vi "GetDatDisplayNm.vi"(8 "error in (no error)":errorcluster caption="entrée d'erreur (pas d'erreur)", 11 "BaseDevice en entrée":refnum<class "BaseDevice.lvclass">) -> (0 "error out":errorcluster caption="sortie d'erreur", 2 "DatDisplayNm":string[](array[string]), 3 "BaseDevice en sortie":refnum<class "BaseDevice.lvclass">)   [LabVIEW 2019, in "BaseDevice.lvclass"]
uses:
  BaseDevice.lvclass
  BaseDevice.lvclass/BaseDevice.ctl
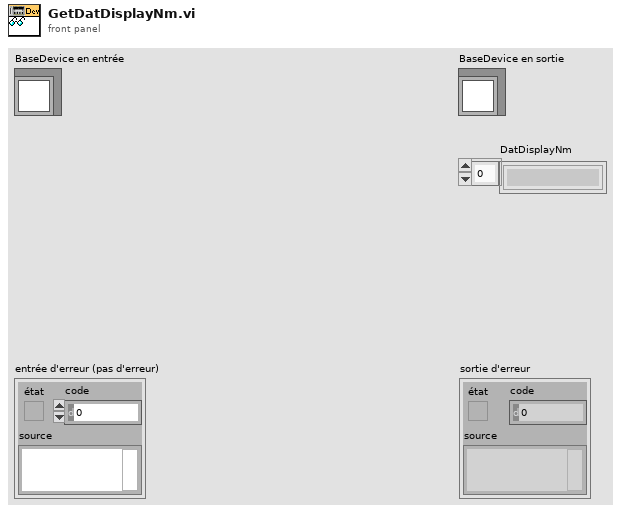
[diagram p1: front panel]
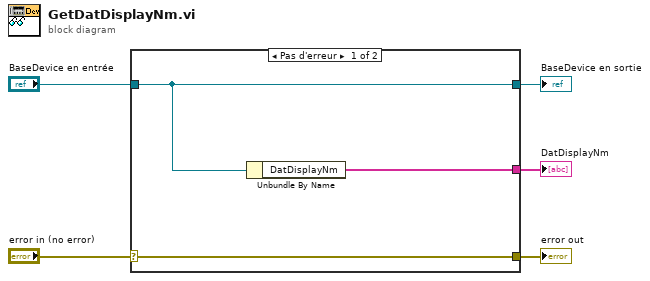
[diagram p0: block diagram]
diagram:
  n1 = case shown="Pas d'erreur" "error in (no error)" {
    selector: "error in (no error)" -> [w8 w9]
    tunnel: [w8 w9] -> w4
    tunnel: [w7 w10] -> w2
    tunnel: "BaseDevice en entrée" -> [w7 w10]
    tunnel: [w6 _] -> w1
    frame No Error {
      n2 = Unbundle By Name(w7) -> ("DatDisplayNm"=w6:string[])
    }
    frame Error {
    }
  }
  "error out" <- w4
  "BaseDevice en sortie" <- w2
  "DatDisplayNm" <- w1
